vi "Configure Digital Input Filter.vi"(5 "Optimize Options (0: Error Vector Magnitude)":i32(ring) items=["Error Vector Magnitude", "Adjacent Channel Power"], 6 "Filter BbT (0.500)":dbl=0.5 min=0.0 max=1.0 step=0.001 format="%.3g", 7 "Filter Alpha (0.500)":dbl=0.5 min=0.0 max=1.0 step=0.001 format="%.3g", 8 "error in (no error)":errorcluster, 9 "User Filter File Name(\"\")":string, 10 "Pre-modulation Filter Type (0: Root Nyquist)":i32(ring) items=["Root Nyquist", "Nyquist", "Gaussian", "IS95", "IS95 EQ", "IS95 MOD", "IS95 MOD EQ", "User Filter", "WCDMA", "Rectangle", "EDGE", "EDGE Wide", "EDGE HSR", "APCO 25 C4FM"], 11 "VISA resource name":refnum<visa-resource-name>) -> (0 "error out":errorcluster, 3 "VISA resource name out":refnum<visa-resource-name>)   [LabVIEW 2018, in "Agilent PSG MXG Series.lvlib"]
doc: "Configures the digital input filters.\n\n<b>Note:</b>\nIt is applicable for N5172B/82B with <b>Option 004</b> only."
uses:
  Agilent PSG MXG Series.lvlib
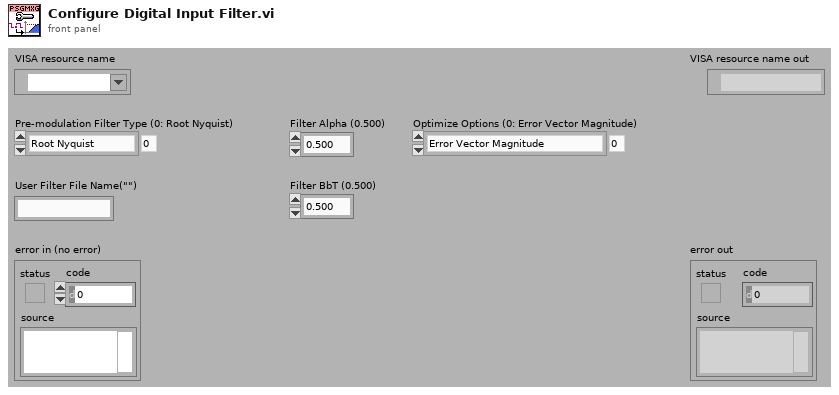
[diagram p1: front panel]
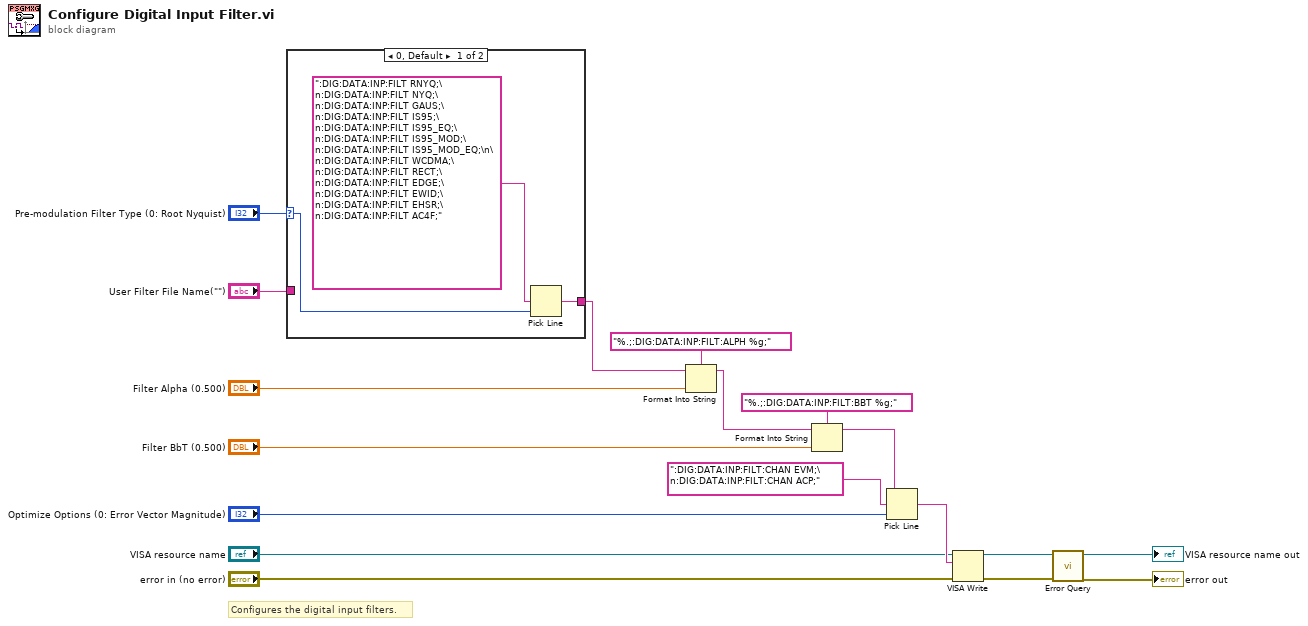
[diagram p0: block diagram]
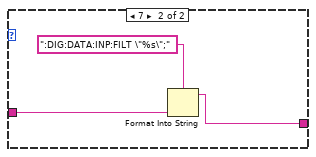
[diagram p2: hidden frame]
diagram:
  # "Configures the digital input filters."
  n1 = case shown="0, Default" "Pre-modulation Filter Type (0: Root Nyquist)" {
    selector: "Pre-modulation Filter Type (0: Root Nyquist)" -> [w20 _]
    tunnel: [w19 w22] -> w2
    tunnel: "User Filter File Name(\"\")" -> [_ w23]
    frame 0, Default {
      n2 = Pick Line(multi-line string=":DIG:DATA:INP:FILT RNYQ;\n:DIG:DATA:INP:FILT NYQ;\n:DIG:DATA:INP:FILT GAUS;\n:DIG:DATA:INP:FILT IS95;\n:DIG:DATA:INP:FILT IS95_EQ;\n:DIG:DATA:INP:FILT IS95_MOD;\n:DIG:DATA:INP:FILT IS95_MOD_EQ;\n\n:DIG:DATA:INP:FILT WCDMA;\n:DIG:DATA:INP:FILT RECT;\n:DIG:DATA:INP:FILT EDGE;\n:DIG:DATA:INP:FILT EWID;\n:DIG:DATA:INP:FILT EHSR;\n:DIG:DATA:INP:FILT AC4F;", line index=w20) -> (output string=w19:string)  [unwired: 1 in]
    }
    frame 7 {
      n3 = Format Into String(format string=":DIG:DATA:INP:FILT \"%s\";", w23) -> (resulting string=w22:string)  [unwired: 2 in, 1 out]
    }
  }
  n4 = Format Into String(format string="%.;:DIG:DATA:INP:FILT:ALPH %g;", initial string=w2, "Filter Alpha (0.500)") -> (resulting string=w16:string)  [unwired: 1 in, 1 out]
  n5 = Format Into String(format string="%.;:DIG:DATA:INP:FILT:BBT %g;", initial string=w16, "Filter BbT (0.500)") -> (resulting string=w11:string)  [unwired: 1 in, 1 out]
  n6 = Pick Line(string ("")=w11, multi-line string=":DIG:DATA:INP:FILT:CHAN EVM;\n:DIG:DATA:INP:FILT:CHAN ACP;", line index="Optimize Options (0: Error Vector Magnitude)") -> (output string=w10:string)
  n7 = VISA Write(VISA resource name="VISA resource name", write buffer=w10, error in (no error)="error in (no error)") -> (VISA resource name out=w7:refnum<visa-resource-name>, error out=w6:errorcluster)  [unwired: 1 out]
  n8 = call "Error Query.vi"("error in (no error)"=w6, "VISA resource name"=w7) -> ("error out"=→"error out":errorcluster, "VISA resource name out"=→"VISA resource name out":refnum<visa-resource-name>)  [unwired: 6 in, 2 out]
